vi "Query USIM SUCI Private Key.vi"(8 "error in (no error)":errorcluster, 9 "Public Key (\"A0\")":string="A0", 10 "SIM Profile (\"SIM1\")":string="SIM1", 11 "VISA resource name":refnum<visa-resource-name>) -> (0 "error out":errorcluster, 2 "Private Key":string, 3 "VISA resource name out":refnum<visa-resource-name>)   [LabVIEW 2020, in "Rohde&Schwarz CMXP Base.lvlib"]
doc: "Queries the subscription concealed identifier (SUCI) home network private key (64-digit hexadecimal number).\n\nAttribute:\n-\n\nRemote-control command:\n[CONFigure:]SIMProfile:USIM:SECurity:HNPPkpair?"
uses:
  <instrlib>/Rohde&Schwarz CMXP Base/Rohde&Schwarz CMXP Base.lvlib
  <instrlib>/Rohde&Schwarz CMXP Base/Private/rsidr_core.llb/rsidr_core.lvlib
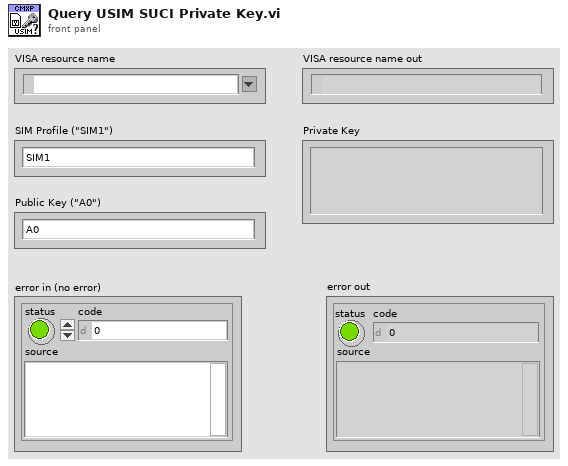
[diagram p1: front panel]
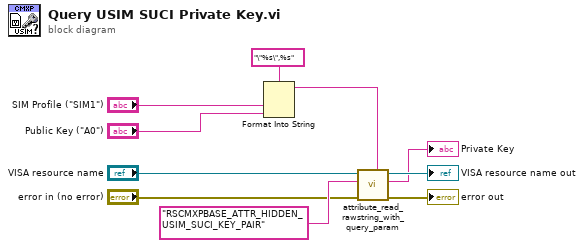
[diagram p0: block diagram]
diagram:
  n1 = Format Into String(format string="\"%s\",%s", "SIM Profile (\"SIM1\")", "Public Key (\"A0\")") -> (resulting string=w8:string)  [unwired: 2 in, 1 out]
  n2 = call <instrlib>:"attribute_read_rawstring_with_query_param.vi"("Query Parameter (None)"=w8, "error in"="error in (no error)", "Attribute ID"="RSCMXPBASE_ATTR_HIDDEN_USIM_SUCI_KEY_PAIR", "VISA resource name"="VISA resource name") -> ("error out"=→"error out":errorcluster, "RawString out"=→"Private Key":string, "VISA resource name out"=→"VISA resource name out":refnum<visa-resource-name>)  [unwired: 5 in]
